vi "Actor Core.vi"(8 "error in":errorcluster, 11 "SimpleExperimentService in":refnum<class "SimpleExperimentService.lvclass">) -> (0 "error out":errorcluster, 3 "Actor out":refnum<class "Actor.lvclass">)   [LabVIEW 2014, in "SimpleExperimentService.lvclass"]
doc: "(<B>Filename</B>: Actor Framework.lvlib:Actor.lvclass:Actor Core.vi)\n\nReceives messages to the actor, reacts to them, and initiates any error handling that may shut the actor down.\n\nDescendant classes may override this VI to append parallel tasks for the actor to complete while it handles messages. Overrides use the Call Parent Method node."
uses:
  SimpleExperimentService.lvclass
  <vilib>/ActorFramework/Actor/Actor.lvclass
  <vilib>/ActorFramework/Actor/Actor.lvclass/Actor.ctl
  <vilib>/ActorFramework/Message Enqueuer/Message Enqueuer.lvclass/Message Enqueuer.ctl
  <vilib>/ActorFramework/Message Enqueuer/Message Priority.ctl
  SimpleExperimentService Messages/Write #Frames Msg/Write #Frames Msg.lvclass/Write #Frames Msg.ctl
  SimpleExperimentService Messages/Write Parameters Array Msg/Write Parameters Array Msg.lvclass/Write Parameters Array Msg.ctl
  ExperimentService/ExperimentService Messages/Set Prefix Msg/Set Prefix Msg.lvclass/Set Prefix Msg.ctl
  <vilib>/ActorFramework/Message Enqueuer/Init from Existing Queue.vi
  <vilib>/ActorFramework/Message Enqueuer/Enqueue.vi
  <vilib>/ActorFramework/Message Priority Queue/Priority Enqueue.vi
  <vilib>/Utility/file.llb/Read From Spreadsheet File (DBL).vi
  <vilib>/ActorFramework/Message Enqueuer/Message Enqueuer.lvclass
  SimpleExperimentService Messages/Write #Frames Msg/Write #Frames Msg.lvclass
  SimpleExperimentService Messages/Write Parameters Array Msg/Write Parameters Array Msg.lvclass
  ExperimentService/ExperimentService Messages/Start Experiment Msg/Start Experiment Msg.lvclass
  ExperimentService/ExperimentService Messages/Set Prefix Msg/Set Prefix Msg.lvclass
  ExperimentService/ExperimentService Messages/Stop Experiment Msg/Stop Experiment Msg.lvclass
  ExperimentService/ExperimentService.lvclass
  Interfaces/Viewable Actor/Viewable Actor.lvclass
  Interfaces/Observable Actor/Observable Actor.lvclass
panel:
  in  "Exp:Add":bool
  in  "Tab":enum32{"Range", "From file"}(tab)
  in  "From":dbl format="%#.5g"
  in  "To":dbl=10.0 format="%#.5g"
  in  "Delta":dbl=1.0 format="%#.5g"
  in  "Path":path
  in  "Type":T1(ring)
  in  "Exp:Clear":bool
  in  "Parameters":i32[](listbox)
  out "Now":dbl format="%#.5g"
  out "Stop":bool=TRUE
  in  "#Frames":u32=10
  in  "Exp:Stop":bool
  in  "Prefix":string
  in  "Exp:Start":bool
  out "Start time":string
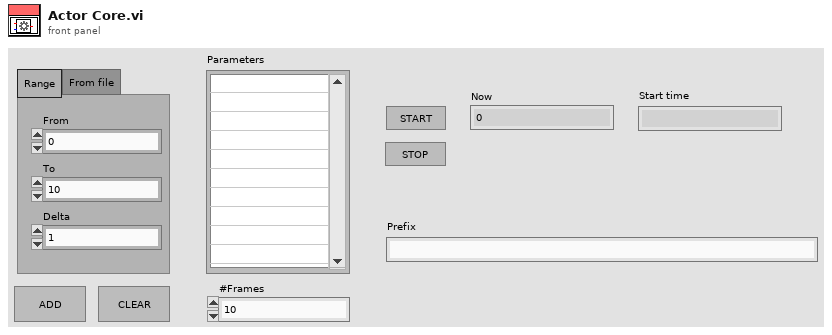
[diagram p1: front panel]
types:
  T1 = enum16{"PARAMETER", "FROM - TO - DELTA", "FROM - TO - N"}
  T2 = typedef "Observable Actor.lvlib/Observable Actor.lvclass/Observer.ctl" = refnum<queue>
  T3 = typedef "Actor Framework.lvlib/Message Enqueuer.lvclass/Message Priority.ctl" = enum16{"Low", "Normal", "High"}
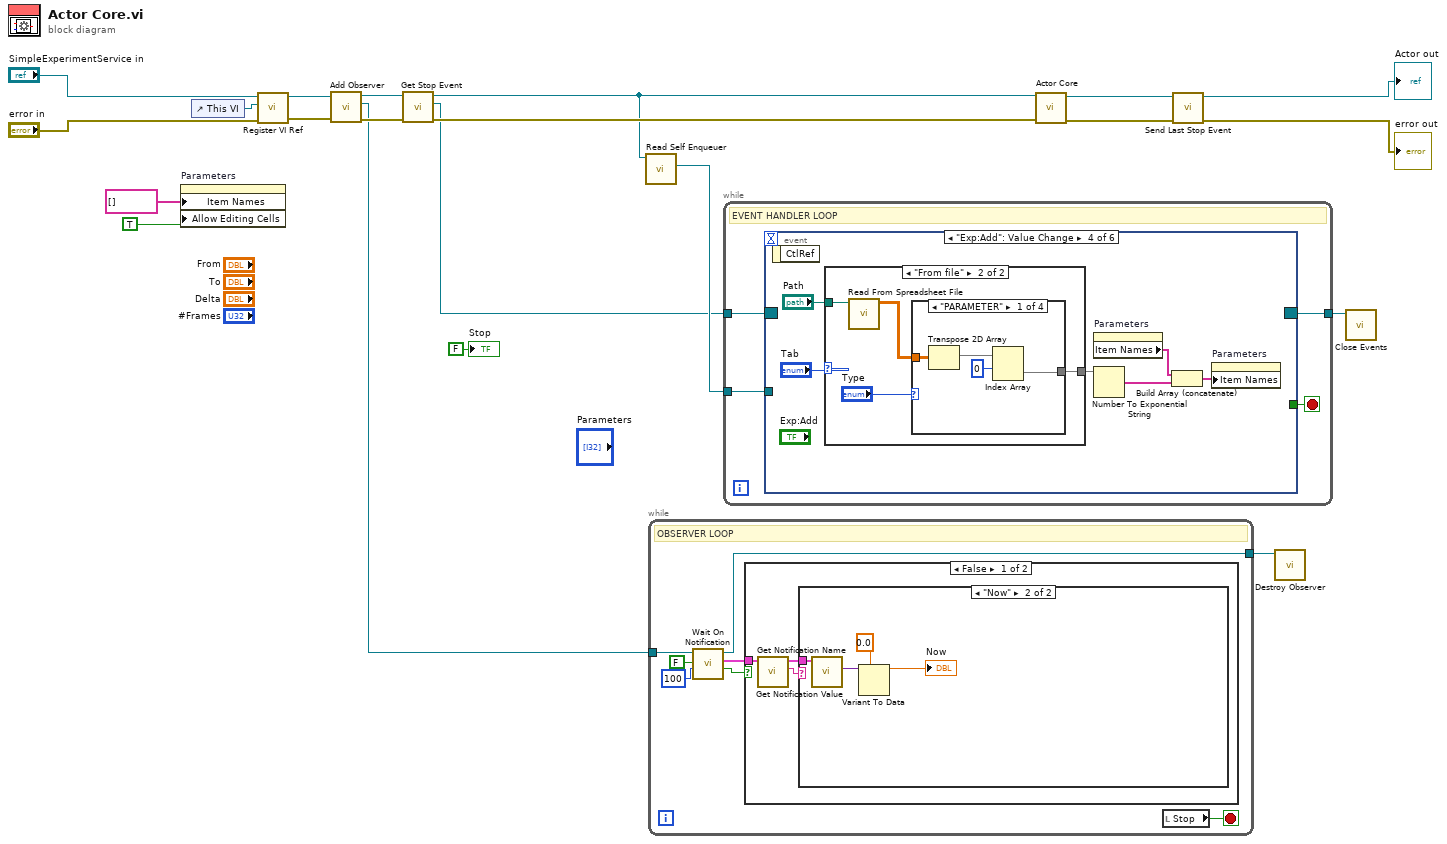
[diagram p0: block diagram]
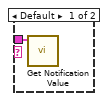
[diagram p2: hidden frame]
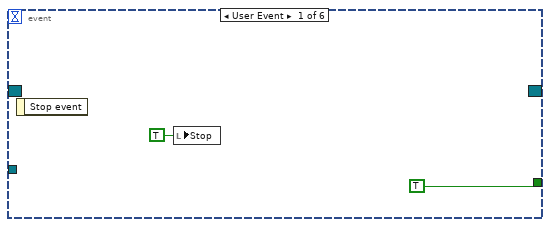
[diagram p4: hidden frame]
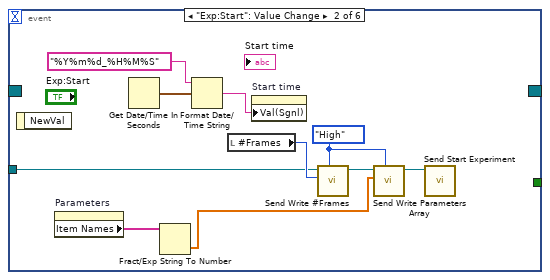
[diagram p5: hidden frame]
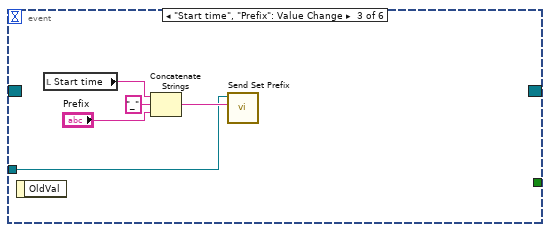
[diagram p6: hidden frame]
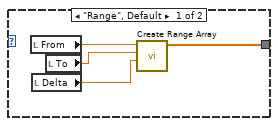
[diagram p7: hidden frame]
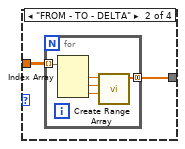
[diagram p8: hidden frame]
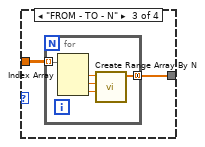
[diagram p9: hidden frame]
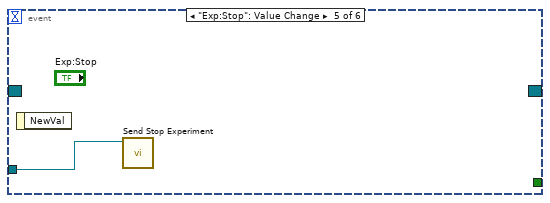
[diagram p11: hidden frame]
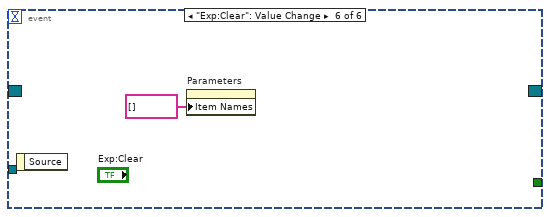
[diagram p12: hidden frame]
diagram:
  n1 = property on="Parameters" class="LstBox (strict)"("Item Names"=string[] [], "Allow Editing Cells"=TRUE) -> ()  [unwired: 2 in, 2 out]
  n2 = control-ref of="This VI"() -> (w21:refnum<vi>)
  n3 = call "Register VI Ref.vi"("error in (no error)"="error in", "VI ref"=w21, "Viewable Actor in"="SimpleExperimentService in") -> ("error out"=w12:errorcluster, "Viewable Actor out"=w8:refnum<class "SimpleExperimentService.lvclass">)  [unwired: 7 in]
  n4 = call-dynamic "Add Observer.vi"("error in (no error)"=w12, "Observable Actor in"=w8) -> ("error out"=w16:errorcluster, "new observer"=w9:T2, "Observable Actor out"=w17:refnum<class "SimpleExperimentService.lvclass">)  [unwired: 7 in]
  n5 = call-dynamic "Get Stop Event.vi"("error in (no error)"=w16, "Observable Actor in"=w17) -> ("error out"=w15:errorcluster, "Events"=w13:refnum<event-registration>, "Observable Actor out"=w3:refnum<class "SimpleExperimentService.lvclass">)  [unwired: 7 in]
  n6 = call <vilib>:"Read Self Enqueuer.vi"("Actor"=w3) -> ("Self Enqueuer"=w20:refnum<class "Message Enqueuer.lvclass">)  [unwired: 10 in]
  n7 = while {
    tunnel: w9 -> [w27]
    tunnel: [w24] -> w10
    stop <- w28 stop-if-true
    # "OBSERVER LOOP"
    n8 = call "Wait On Notification.vi"("timeout in ms (-1)"=100, "ignore previous (F)"=FALSE, "observer in"=w27) -> ("timed out?"=w22:bool, "notification"=w23:cluster{"value":variant, "name":string}, "observer out"=w24:T2)  [unwired: 5 in, 1 out]
    n9 = case shown="False" w22 {
      tunnel: w23 -> [w31 _]
      frame False {
        n10 = call "Get Notification Name.vi"("notification in"=w31) -> ("name"=w29:string, "notification out"=w30:cluster{"value":variant, "name":string})  [unwired: 9 in]
        n11 = case shown="\"Now\"" w29 {
          tunnel: w30 -> [w32 w35]
          frame Default {
            n12 = call "Get Notification Value.vi"("notification in"=w32) -> ()  [unwired: 7 in, 2 out]
          }
          frame "Now" {
            n13 = call "Get Notification Value.vi"("notification in"=w35) -> ("data"=w36:variant)  [unwired: 7 in, 1 out]
            n14 = Variant To Data(type=0.0, Variant=w36) -> (data=→"Now":dbl)  [unwired: 1 in, 1 out]
          }
        }
      }
      frame True {
      }
    }
    n15 = local read "Stop"() -> (w28:bool)
  }
  n16 = while {
    tunnel: w13 -> [w40]
    tunnel: w20 -> [w39]
    tunnel: [w38] -> w14
    stop <- w37 stop-if-true
    # "EVENT HANDLER LOOP"
    n17 = event shown="[3] \"Exp:Add\": Value Change" {
      selector: w40 -> [_ _ _ _ _ _]
      dyn-events: [_ _ _ _ _ _] -> w38
      timeout: _ -> [_ _ _ _ _ _]
      tunnel: w39 -> [_ w48 w53 _ w90 _]
      tunnel: [TRUE _ _ _ _ _] -> w37
      event User Event {
        n18 = event-data() -> ()  [unwired: 1 in, 1 out]
        n19 = local write "Stop"(TRUE ("Stop")) -> ()
      }
      event "Exp:Start": Value Change {
        w46 = Message_Priority."High" ("Message Priority (Normal)")
        n20 = event-data() -> ()  [unwired: 1 in, 1 out]
        n21 = property on="Parameters" class="LstBox (strict)"() -> ("Item Names"=w44:string[])  [unwired: 2 in, 2 out]
        n22 = Get Date/Time In Seconds() -> (seconds since 1Jan1904=w52:timestamp)
        n23 = Fract/Exp String To Number(string=w44) -> (number=w43:dbl[])  [unwired: 3 in, 1 out]
        n24 = Format Date/Time String(time format string (%c)="%Y%m%d_%H%M%S", seconds (now)=w52) -> (date/time string=w50:string)  [unwired: 1 in]
        n25 = local read "#Frames"() -> (w49:u32)
        n26 = property on="Start time" class="Str"("Val(Sgnl)"=w50) -> ()  [unwired: 2 in, 2 out]
        n27 = call "Send Write #Frames.vi"("Message Priority (Normal)"=w46, "#Frames"=w49, "Message Enqueuer"=w48) -> ("Message Enqueuer out"=w47:refnum<class "Message Enqueuer.lvclass">)  [unwired: 7 in, 1 out]
        n28 = call "Send Write Parameters Array.vi"("Message Priority (Normal)"=w46, "Parameters Array"=w43, "Message Enqueuer"=w47) -> ("Message Enqueuer out"=w45:refnum<class "Message Enqueuer.lvclass">)  [unwired: 7 in, 1 out]
        n29 = call "Send Start Experiment.vi"("Message Enqueuer"=w45) -> ()  [unwired: 9 in, 2 out]
      }
      event "Start time", "Prefix": Value Change {
        n30 = event-data() -> ()  [unwired: 1 in, 1 out]
        n31 = local read "Start time"() -> (w55:string)
        n32 = Concatenate Strings(w55, "_" ("string"), "Prefix") -> (w54:string)
        n33 = call "Send Set Prefix.vi"("Prefix"=w54, "Message Enqueuer"=w53) -> ()  [unwired: 8 in, 2 out]
      }
      event "Exp:Add": Value Change {
        n34 = event-data() -> ()  [unwired: 1 in, 1 out]
        n35 = case shown="\"From file\"" "Tab" {
          tunnel: [w67 w68] -> w61
          tunnel: "Path" -> [_ w70]
          frame "Range", Default {
            n36 = local read "From"() -> (w66:dbl)
            n37 = local read "Delta"() -> (w64:dbl)
            n38 = local read "To"() -> (w65:dbl)
            n39 = call "Create Range Array.vi"("Delta"=w64, "To"=w65, "From"=w66) -> ("Array"=w67:dbl[])  [unwired: 8 in]
          }
          frame "From file" {
            n40 = call-poly <vilib>:"Read From Spreadsheet File.vi"("file path (dialog if empty)"=w70) -> ("all rows"=w69:dbl[][])  [unwired: 6 in, 4 out]
            n41 = case shown="\"PARAMETER\"" "Type" {
              tunnel: w69 -> [w75 w77 w84 _]
              tunnel: [w72 w76 w83 _] -> w68
              frame "PARAMETER" {
                n42 = Transpose 2D Array(2D array=w75) -> (transposed array=w74:dbl[][])
                n43 = Index Array(array=w74, index (row)=0) -> (element=w72:dbl[])  [unwired: 1 in]
              }
              frame "FROM - TO - DELTA" {
                n44 = for {
                  tunnel: w77 -> [w82] mode=indexing
                  tunnel: [w78] -> w76 mode=concatenating
                  n45 = Index Array(array=w82) -> (element #1=w81:dbl, element #2=w80:dbl, element #3=w79:dbl)  [unwired: 3 in]
                  n46 = call "Create Range Array.vi"("Delta"=w79, "To"=w80, "From"=w81) -> ("Array"=w78:dbl[])  [unwired: 8 in]
                }
              }
              frame "FROM - TO - N" {
                n47 = for {
                  tunnel: w84 -> [w89] mode=indexing
                  tunnel: [w85] -> w83 mode=concatenating
                  n48 = Index Array(array=w89) -> (element #1=w88:dbl, element #2=w87:dbl, element #3=w86:dbl)  [unwired: 3 in]
                  n49 = call "Create Range Array By N.vi"("N"=w86, "To"=w87, "From"=w88) -> ("Array"=w85:dbl[])  [unwired: 8 in]
                }
              }
              frame Default {
              }
            }
          }
        }
        n50 = property on="Parameters" class="LstBox (strict)"() -> ("Item Names"=w58:string[])  [unwired: 2 in, 2 out]
        n51 = Number To Exponential String(number=w61) -> (E-format string=w59:string[])  [unwired: 3 in]
        n52 = Build Array (concatenate)(w58, w59) -> (w60:string[])
        n53 = property on="Parameters" class="LstBox (strict)"("Item Names"=w60) -> ()  [unwired: 2 in, 2 out]
      }
      event "Exp:Stop": Value Change {
        n54 = event-data() -> ()  [unwired: 1 in, 1 out]
        n55 = call "Send Stop Experiment.vi"("Message Enqueuer"=w90) -> ()  [unwired: 9 in, 2 out]
      }
      event "Exp:Clear": Value Change {
        n56 = event-data() -> ()  [unwired: 1 in, 1 out]
        n57 = property on="Parameters" class="LstBox (strict)"("Item Names"=string[] []) -> ()  [unwired: 2 in, 2 out]
      }
    }
  }
  n58 = call-parent "Actor Core.vi"("error in"=w15, "Actor in"=w3) -> ("error out"=w18:errorcluster, "Actor out"=w19:refnum<class "Actor.lvclass">)  [unwired: 8 in]
  n59 = call "Send Last Stop Event.vi"("error in (no error)"=w18, "Actor in"=w19) -> ("error out"=→"error out":errorcluster, "Actor  out"=→"Actor out":refnum<class "Actor.lvclass">)  [unwired: 8 in]
  n60 = call "Destroy Observer.vi"("observer in"=w10) -> ()  [unwired: 11 in]
  n61 = call "Close Events.vi"("events"=w14) -> ()  [unwired: 11 in]
  "Stop" <- FALSE ("Stop")
